vi "Add Major Frame.vi"(6 "minorFrameRefs":refnum<k24>[](array[refnum]), 7 "minorFramePeriod":i32, 8 "error in":errorcluster, 9 "minorFrameNames":string[](array[string]), 10 "name":string, 11 "channel in":refnum<k24>) -> (0 "error out":errorcluster, 2 "new major frame":refnum<k24>, 3 "channel out":refnum<k24>)   [LabVIEW 2020, in "AIM_1553_Parameter_ni.lvlib"]
uses:
  AIM_1553_Parameter_ni.lvlib
  C:/Users/Administrator/Desktop/GIT/Ballard-Arinc-429-XML-Generator/Source/Assemblies/Aim_1553_Parameter_ni/bin/Debug/AIM_1553_Parameter_ni.dll
  Assemblies/Aim_1553_Parameter_ni/bin/Debug/AIM_1553_Parameter_ni.dll
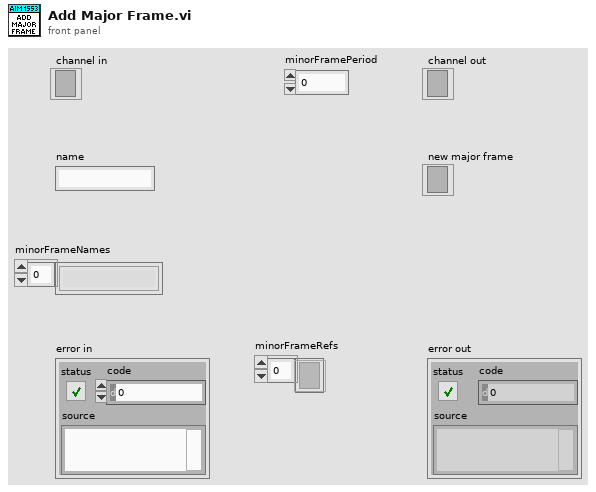
[diagram p1: front panel]
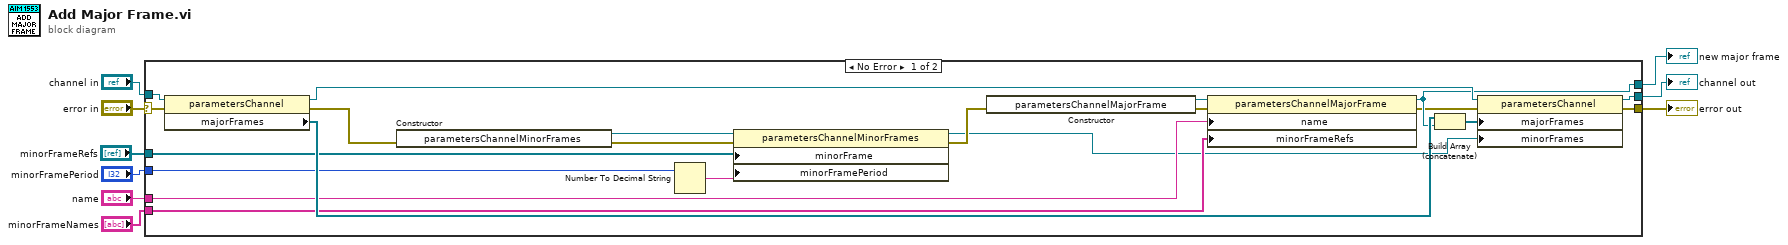
[diagram p0: block diagram]
diagram:
  n1 = case shown="No Error" "error in" {
    selector: "error in" -> [w29 w31]
    tunnel: [w26 w32] -> w9
    tunnel: [w25 w31] -> w8
    tunnel: "channel in" -> [w30 w32]
    tunnel: [w20 _] -> w4
    tunnel: "name" -> [w21 _]
    tunnel: "minorFrameNames" -> [w18 _]
    tunnel: "minorFramePeriod" -> [w16 _]
    tunnel: "minorFrameRefs" -> [w14 _]
    frame No Error {
      n2 = property class="parametersChannel"(reference=w30, error in=w29) -> (reference out=w27:refnum<k24>, error out=w13:errorcluster, "majorFrames"=w28:refnum<k24>[])
      n3 = constructor class="parametersChannelMinorFrames"(error in=w13) -> (reference out=w11:refnum<k24>, error out=w12:errorcluster)  [unwired: 2 in, 1 out]
      n4 = Number To Decimal String(number=w16) -> (decimal integer string=w17:string)  [unwired: 1 in]
      n5 = property class="parametersChannelMinorFrames"(reference=w11, error in=w12, "minorFrame"=w14, "minorFramePeriod"=w17) -> (reference out=w10:refnum<k24>, error out=w15:errorcluster)
      n6 = constructor class="parametersChannelMajorFrame"(error in=w15) -> (reference out=w22:refnum<k24>, error out=w23:errorcluster)  [unwired: 2 in, 1 out]
      n7 = property class="parametersChannelMajorFrame"(reference=w22, error in=w23, "name"=w21, "minorFrameRefs"=w18) -> (reference out=w20:refnum<k24>, error out=w19:errorcluster)
      n8 = Build Array (concatenate)(w28, w20) -> (w24:refnum<k24>[])
      n9 = property class="parametersChannel"(reference=w27, error in=w19, "majorFrames"=w24, "minorFrames"=w10) -> (reference out=w26:refnum<k24>, error out=w25:errorcluster)
    }
    frame Error {
    }
  }
  "channel out" <- w9
  "error out" <- w8
  "new major frame" <- w4
